vi "Find Sparks with RF Envelope.vi"(3 "RF Hammer Duration (S)":u32, 4 "Min Spark Length":i32=5000, 5 "error in (no error)":errorcluster, 6 "Waveform":dbl[](array[numeric])) -> (0 "error out":errorcluster, 2 "Spark Indicies":i32[](array[numeric]))   [LabVIEW 2013]
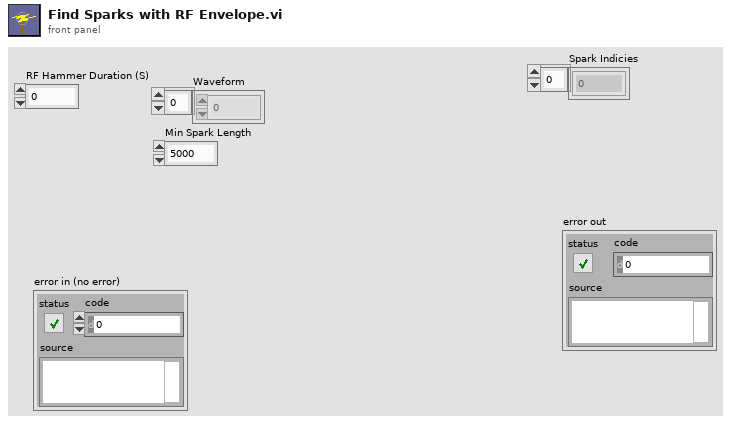
[diagram p1: front panel]
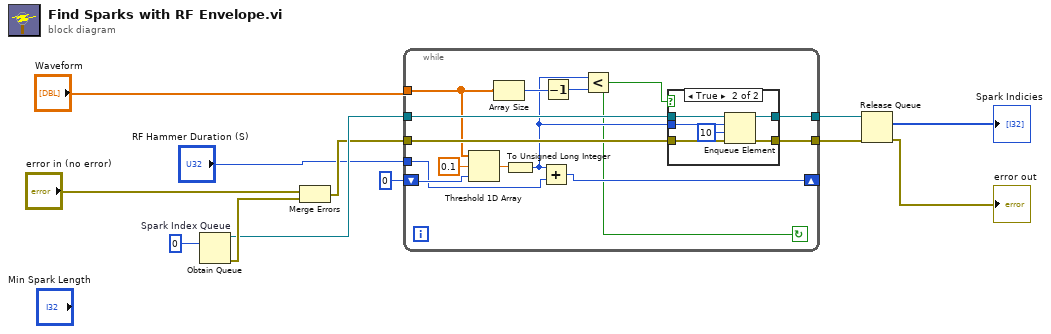
[diagram p0: block diagram]
diagram:
  n1 = Obtain Queue "Spark Index Queue"(element data type=0 ("# Cluster Levels")) -> (queue out=w7:refnum<queue>, error out=w11:errorcluster)  [unwired: 4 in, 1 out]
  n2 = Merge Errors("error in (no error)", w11) -> (w6:errorcluster)
  n3 = while {
    tunnel: "Waveform" -> [w18]
    shift-right: [w15] -> _
    shift-left: 0 ("start index (0)") -> [w21]
    tunnel: w7 -> [w26]
    tunnel: w6 -> [w25]
    tunnel: [w24] -> w5
    tunnel: [w23] -> w4
    tunnel: "RF Hammer Duration (S)" -> [w19]
    stop <- w13 continue-if-true
    n4 = Threshold 1D Array(1:w21, 2:0.1 ("threshold y"), 3:w18) -> (0:w22:dbl)
    n5 = Array Size(array=w18) -> (size(s)=w17:i32)
    n6 = To Unsigned Long Integer(number=w22) -> (unsigned 32bit integer=w14:u32)
    n7 = Add(x=w14, y=w19) -> (x+y=w15:u32)
    n8 = Decrement(x=w17) -> (x-1=w16:i32)
    n9 = Less?(x=w14, y=w16) -> (x < y?=w13:bool)
    n10 = case shown="True" w13 {
      tunnel: w26 -> [w28 w34]
      tunnel: w25 -> [w27 w33]
      tunnel: [w28 w32] -> w24
      tunnel: [w27 w31] -> w23
      tunnel: w14 -> [_ w30]
      frame False {
      }
      frame True {
        n11 = Enqueue Element(queue=w34, element=w30, timeout in ms (-1)=10, error in (no error)=w33) -> (queue out=w32:refnum<queue>, error out=w31:errorcluster)  [unwired: 1 out]
      }
    }
  }
  n12 = Release Queue(queue=w5, error in (no error)=w4) -> (remaining elements=→"Spark Indicies":i32[], error out=→"error out":errorcluster)  [unwired: 1 in, 1 out]
